vi "Create AXI4-Stream Resources.vi"(10 "RX CLIP Resources":T1, 11 "TX CLIP Resources":T2) -> (2 "RX niInstr AXI4-Stream Reader FXP64x1 v1 FPGA out":refnum<class "niInstr AXI4-Stream Reader FXP64x1 v1 FPGA.lvclass">, 3 "TX niInstr AXI4-Stream Reader FXP64x1 v1 FPGA out":refnum<class "niInstr AXI4-Stream Writer FXP64x1 v1 FPGA.lvclass">)   [LabVIEW 2016, in "Aurora Stream (NI 6592R) (FPGA).lvlib"]
doc: "Creates an AXI4-Stream Address Space Collection with the selected <b>CLIP Resources</b> at the appropriate offsets.\n\n<B>Input Parameters</B>\n\n<B>RX CLIP Resources</B> specifies the CLIP resources to use for the RX portion of AXI4-Stream.\n\n<B>TX CLIP Resources</B> specifies the CLIP resources to use for the TX portion of AXI4-Stream.\n\n<B>Output Parameters</B>\n\n<B>RX niInstr AXI4-Stream Reader FXP64x1 v1 FPGA out</B> passes a reference to the newly-created RX AXI4-Stream Reader to the next VI.\n\n<B>TX niInstr AXI4-Stream Reader FXP64x1 v1 FPGA out</B> passes a reference to the newly-created TX AXI4-Stream Writer to the next VI."
uses:
  Aurora Stream (NI 6592R) (FPGA).lvlib
  <instrlib>/_niInstr/CLIP Adapters/v1/FPGA/AXI4-Stream/Writer FXP64x1/niInstr AXI4-Stream Writer FXP64x1 v1 FPGA.lvclass
  C:/Program Files (x86)/National Instruments/LabVIEW 2016/instr.lib/_niInstr/CLIP Adapters/v1/FPGA/AXI4-Stream/Writer/niInstr AXI4-Stream Writer v1 FPGA.lvclass
  <instrlib>/_niInstr/CLIP Adapters/v1/FPGA/AXI4-Stream/Reader FXP64x1/niInstr AXI4-Stream Reader FXP64x1 v1 FPGA.lvclass
  <instrlib>/_niInstr/CLIP Adapters/v1/FPGA/AXI4-Stream/Writer FXP64x1/Public/Create Resources.vi
  <instrlib>/_niInstr/CLIP Adapters/v1/FPGA/AXI4-Stream/Writer/Public/Enable TREADY.vi
  <instrlib>/_niInstr/CLIP Adapters/v1/FPGA/AXI4-Stream/Reader FXP64x1/Public/Create Resources.vi
  <instrlib>/_niInstr/CLIP Adapters/v1/FPGA/AXI4-Stream/Reader/niInstr AXI4-Stream Reader v1 FPGA.lvclass
  <instrlib>/_niInstr/CLIP Adapters/v1/FPGA/AXI4-Stream/Writer/niInstr AXI4-Stream Writer v1 FPGA.lvclass
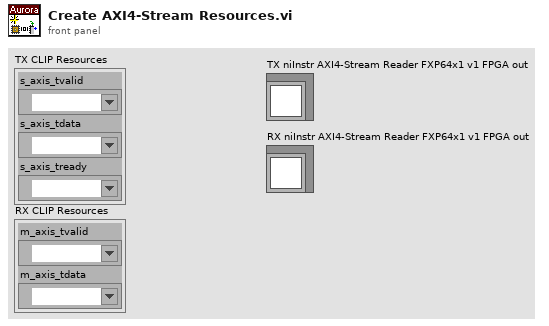
[diagram p1: front panel]
types:
  T1 = cluster{"m_axis_tvalid":refnum<k21>, "m_axis_tdata":refnum<k21>}
  T2 = cluster{"s_axis_tvalid":refnum<k21>, "s_axis_tdata":refnum<k21>, "s_axis_tready":refnum<k21>}
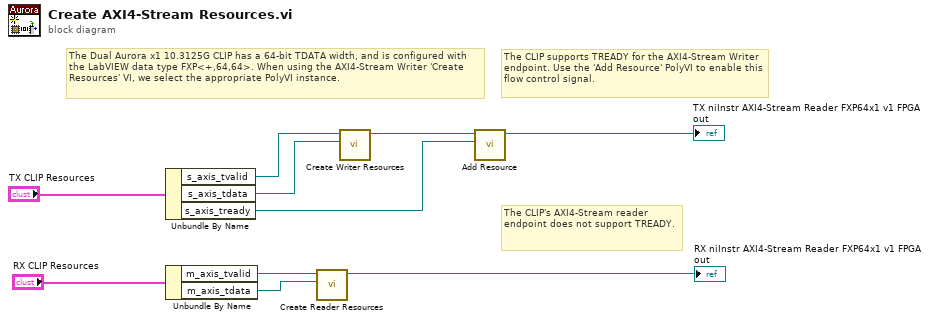
[diagram p0: block diagram]
diagram:
  # "The CLIP's AXI4-Stream reader endpoint does not support TREADY."
  # "The CLIP supports TREADY for the AXI4-Stream Writer endpoint. Use the 'Add Resource' PolyVI to enable this flow control signal."
  # "The Dual Aurora x1 10.3125G CLIP has a 64-bit TDATA width, and is configured with the LabVIEW data type FXP<+,64,64>. When using the AXI4-Stream Writer 'Create Resources' VI, we select the appropriate PolyVI instance."
  n1 = Unbundle By Name("TX CLIP Resources") -> ("s_axis_tvalid"=w6:refnum<k21>, "s_axis_tdata"=w5:refnum<k21>, "s_axis_tready"=w4:refnum<k21>)
  n2 = Unbundle By Name("RX CLIP Resources") -> ("m_axis_tvalid"=w2:refnum<k21>, "m_axis_tdata"=w1:refnum<k21>)
  n3 = call-poly <instrlib>:"Create Reader Resources.vi"("m_axis_tdata"=w1, "m_axis_tvalid"=w2) -> ("niInstr AXI4-Stream Reader FXP64x1 v1 FPGA out"=→"RX niInstr AXI4-Stream Reader FXP64x1 v1 FPGA out":refnum<class "niInstr AXI4-Stream Reader FXP64x1 v1 FPGA.lvclass">)  [unwired: 9 in]
  n4 = call-poly <instrlib>:"Create Writer Resources.vi"("s_axis_tdata"=w5, "s_axis_tvalid"=w6) -> ("niInstr AXI4-Stream Writer FXP64x1 v1 FPGA out"=w10:refnum<class "niInstr AXI4-Stream Writer FXP64x1 v1 FPGA.lvclass">)  [unwired: 9 in]
  n5 = call-poly <instrlib>:"Add Resource.vi"("s_axis_tready"=w4, "niInstr AXI4-Stream Writer v1 FPGA in"=w10) -> ("niInstr AXI4-Stream Writer v1 FPGA out"=→"TX niInstr AXI4-Stream Reader FXP64x1 v1 FPGA out":refnum<class "niInstr AXI4-Stream Writer FXP64x1 v1 FPGA.lvclass">)  [unwired: 9 in]
